vi "Negative_To_Positive.vi"(1 "Number":i32) -> (0 "Positive":i32)   [LabVIEW 2021]
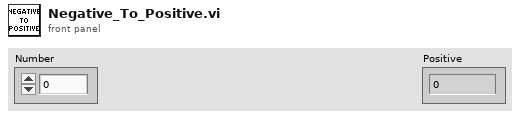
[diagram p1: front panel]
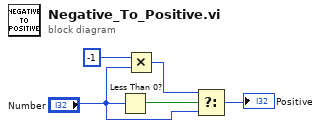
[diagram p0: block diagram]
diagram:
  n1 = Less Than 0?(x="Number") -> (x < 0?=w5:bool)
  n2 = Multiply(x=-1, y="Number") -> (x*y=w3:i32)
  n3 = Select(t=w3, s=w5, f="Number") -> (s? t:f=→"Positive":i32)
